vi "Request Message Loop.vi"(8 "error in (no error)":errorcluster, 11 "Message Queues":T1) -> (0 "error out":errorcluster)   [LabVIEW 2023, in "Weather Request Loop.lvlib"]
doc: "A message handler for sending HTTP requests and parsing the response headers. If needed, the handler will prompt the user to log in."
uses:
  Weather Request Loop.lvlib
  support/Message Queue/All Message Queues.ctl
  support/Message Queue/Message Cluster.ctl
  Request Data.ctl
  <vilib>/httpClient/ClientHandle.ctl
  Response Data.ctl
  support/Message Queue/Weather Message Queue.lvlib
  <vilib>/httpClient/LabVIEWHTTPClient.lvlib
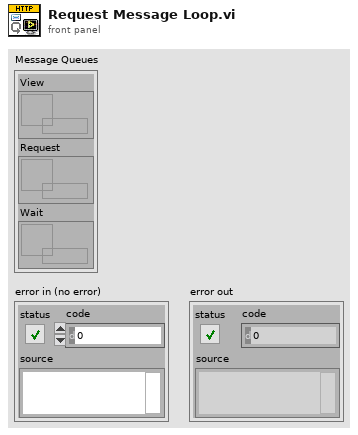
[diagram p1: front panel]
types:
  T1 = typedef "Weather Message Queue.lvlib/All Message Queues.ctl" = cluster{"View":refnum<queue>, "Request":refnum<queue>, "Wait":refnum<queue>}
  T2 = typedef "Weather Request Loop.lvlib/Request Data.ctl" = cluster{"client handle":T3, "URL":string, "Content-Type":string, "Timeout":i32}
  T3 = typedef "LabVIEWHTTPClient.lvlib/ClientHandle.ctl" = refnum<k1>
  T4 = typedef "Weather Request Loop.lvlib/Response Data.ctl" = cluster{"Response Code":u16, "Body":string, "Headers":variant, "error":errorcluster}
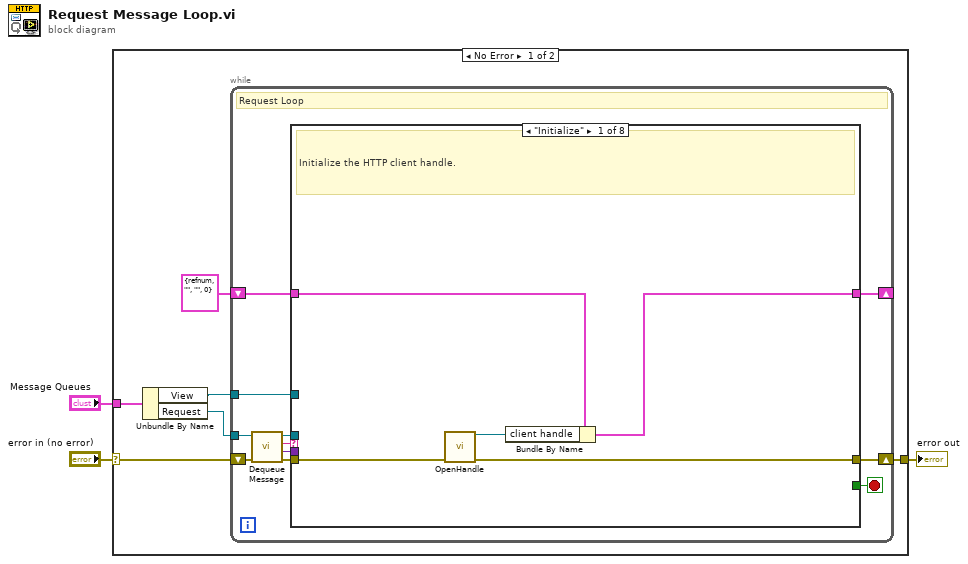
[diagram p0: block diagram]
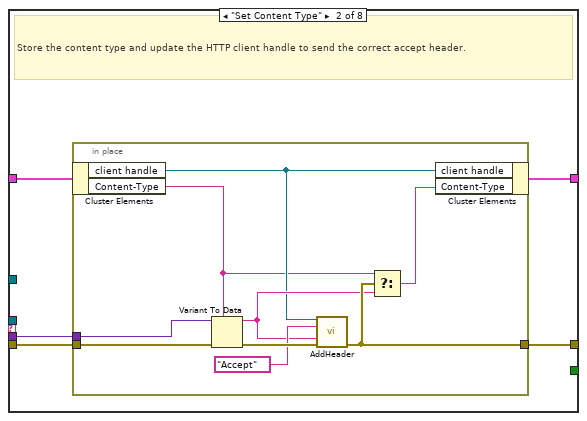
[diagram p2: hidden frame]
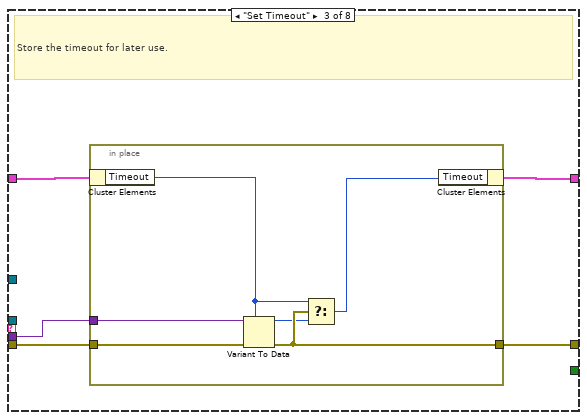
[diagram p3: hidden frame]
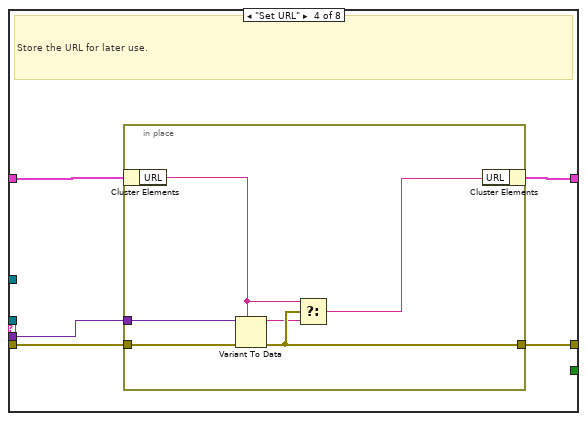
[diagram p4: hidden frame]
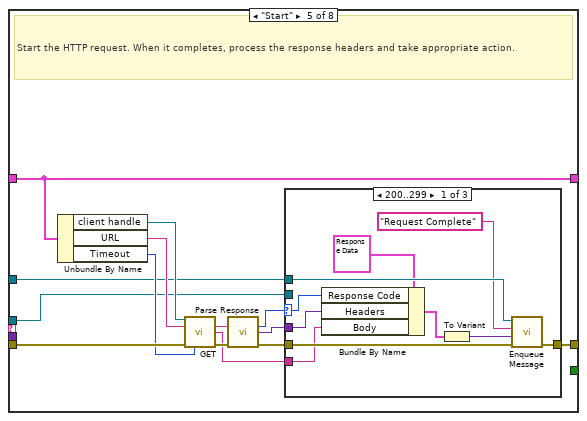
[diagram p5: hidden frame]
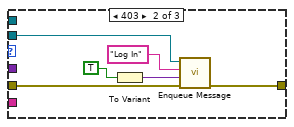
[diagram p6: hidden frame]
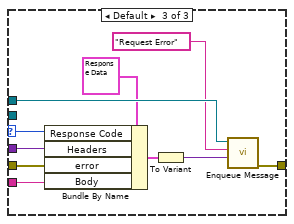
[diagram p7: hidden frame]
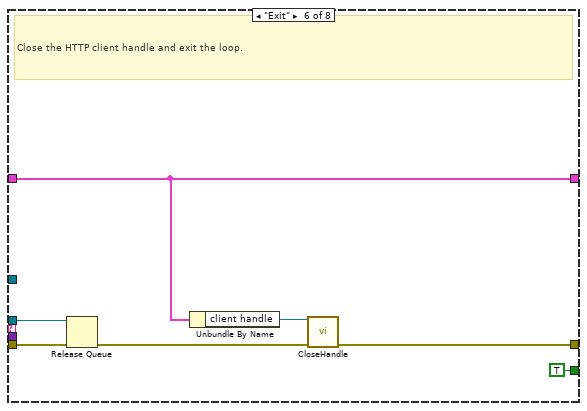
[diagram p8: hidden frame]
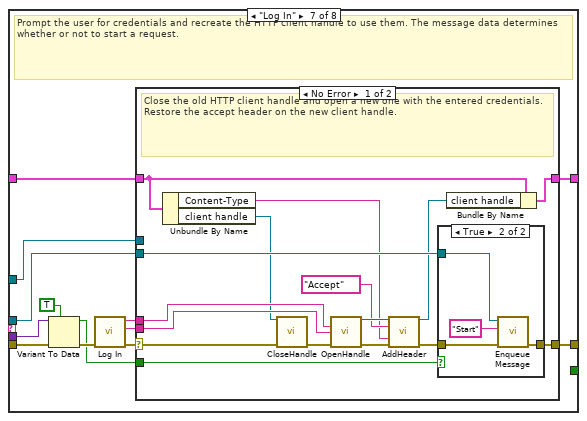
[diagram p9: hidden frame]
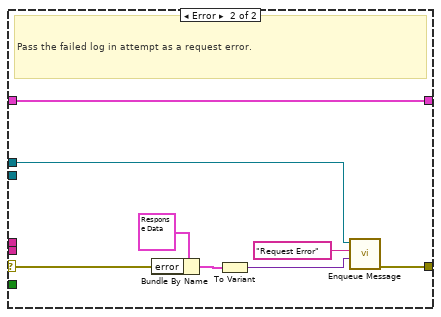
[diagram p11: hidden frame]
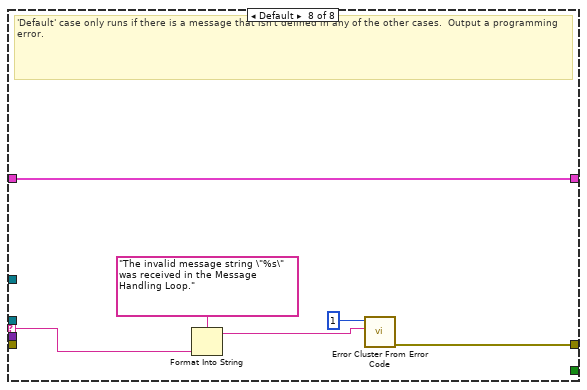
[diagram p12: hidden frame]
diagram:
  n1 = case shown="No Error" "error in (no error)" {
    selector: "error in (no error)" -> [w8 w157]
    tunnel: "Message Queues" -> [w9 _]
    tunnel: [w7 w157] -> w1
    frame No Error {
      n2 = Unbundle By Name(w9) -> ("View"=w6:refnum<queue>, "Request"=w5:refnum<queue>)
      n3 = while {
        shift-right: [w12] -> w7
        shift-left: w8 -> [w19]
        tunnel: w6 -> [w10]
        tunnel: w5 -> [w20]
        shift-right: [w13] -> _
        shift-left: T2 {"client handle"=refnum, "URL"="", "Content-Type"="", "Timeout"=0} ("Request Data") -> [w14]
        stop <- w11 stop-if-true
        # "Request Loop"
        n4 = call "Dequeue Message.vi"("error in (no error)"=w19, "Message Queue"=w20) -> ("error out"=w16:errorcluster, "Message Data"=w15:variant, "Message"=w18:string, "dup Message Queue"=w17:refnum<queue>)  [unwired: 6 in]
        n5 = case shown="\"Initialize\"" w18 {
          selector: w18 -> [_ _ _ _ _ _ _ w151]
          tunnel: w17 -> [_ _ _ _ w63 w102 w113 _]
          tunnel: w16 -> [w25 w30 w44 w55 w75 w108 w121 _]
          tunnel: w15 -> [_ w29 w42 w53 _ _ w111 _]
          tunnel: w14 -> [w24 w27 w41 w52 w74 w105 w117 w156]
          tunnel: [w22 w26 w40 w51 w74 w105 w116 w156] -> w13
          tunnel: [w21 w28 w43 w54 w67 w106 w119 w152] -> w12
          tunnel: [_ _ _ _ _ TRUE _ _] -> w11
          tunnel: w10 -> [_ _ _ _ w65 _ w118 _]
          frame "Initialize" {
            # "Initialize the HTTP client handle."
            n6 = call <vilib>:"OpenHandle.vi"("error in (no error)"=w25) -> ("client handle out"=w23:T3, "error out"=w21:errorcluster)  [unwired: 13 in]
            n7 = Bundle By Name(cluster=w24, "client handle"=w23) -> (w22:T2)
          }
          frame "Set Content Type" {
            # "Store the content type and update the HTTP client handle to send the correct accept header."
            n8 = in-place {
              in-place-border: w30 -> [w39]
              in-place-border: w29 -> [w37]
              in-place-border: [w35] -> w28
              n9 = in-place-cluster #1(w27) -> ("client handle"=w32:T3, "Content-Type"=w31:string)
              n10 = Variant To Data(error in=w39, type=w31, Variant=w37) -> (data=w34:string, error out=w38:errorcluster)
              n11 = call <vilib>:"AddHeader.vi"("client handle"=w32, "header"="Accept", "value"=w34, "error in (no error)"=w38) -> ("error out"=w35:errorcluster)  [unwired: 10 in, 1 out]
              n12 = Select(t=w31, s=w35, f=w34) -> (s? t:f=w33:string)
              n13 = in-place-cluster #1("client handle"=w32, "Content-Type"=w33) -> (w26:T2)
            }
          }
          frame "Set Timeout" {
            # "Store the timeout for later use."
            n14 = in-place {
              in-place-border: w44 -> [w50]
              in-place-border: [w49] -> w43
              in-place-border: w42 -> [w48]
              n15 = in-place-cluster #2(w41) -> ("Timeout"=w46:i32)
              n16 = Variant To Data(error in=w50, type=w46, Variant=w48) -> (data=w47:i32, error out=w49:errorcluster)
              n17 = Select(t=w46, s=w49, f=w47) -> (s? t:f=w45:i32)
              n18 = in-place-cluster #2("Timeout"=w45) -> (w40:T2)
            }
          }
          frame "Set URL" {
            # "Store the URL for later use."
            n19 = in-place {
              in-place-border: w55 -> [w61]
              in-place-border: [w60] -> w54
              in-place-border: w53 -> [w59]
              n20 = in-place-cluster #3(w52) -> ("URL"=w57:string)
              n21 = Variant To Data(error in=w61, type=w57, Variant=w59) -> (data=w58:string, error out=w60:errorcluster)
              n22 = Select(t=w57, s=w60, f=w58) -> (s? t:f=w56:string)
              n23 = in-place-cluster #3("URL"=w56) -> (w51:T2)
            }
          }
          frame "Start" {
            # "Start the HTTP request. When it completes, process the response headers and take appropriate action."
            n24 = Unbundle By Name(w74) -> ("client handle"=w73:T3, "URL"=w72:string, "Timeout"=w71:i32)
            n25 = call <vilib>:"GET.vi"("client handle"=w73, "url"=w72, "error in (no error)"=w75, "timeout (10000)"=w71) -> ("headers"=w70:string, "body"=w62:string, "error out"=w69:errorcluster)  [unwired: 8 in, 1 out]
            n26 = call "Parse Response.vi"("Headers"=w70, "error in (no error)"=w69) -> ("Response code"=w66:u16, "Parsed headers"=w64:variant, "error out"=w68:errorcluster)  [unwired: 11 in]
            n27 = case shown="200..299" w66 {
              selector: w66 -> [w81 _ w95]
              tunnel: w68 -> [w85 w91 w97]
              tunnel: [w84 w90 w101] -> w67
              tunnel: w65 -> [w83 _ w100]
              tunnel: w64 -> [w80 _ w96]
              tunnel: w63 -> [_ w89 _]
              tunnel: w62 -> [w76 _ w92]
              frame 200..299 {
                n28 = Bundle By Name(cluster=T4 {"Response Code"=0, "Body"="", "Headers"=variant, "error"={"status"=FALSE, "code"=0, "source"=""}} ("Response Data"), "Response Code"=w81, "Headers"=w80, "Body"=w76) -> (w79:T4)
                n29 = To Variant(anything=w79) -> (Variant=w78:variant)
                n30 = call "Enqueue Message.vi"("error in (no error)"=w85, "Message Data"=w78, "Message"="Request Complete", "Message Queue"=w83) -> ("error out"=w84:errorcluster)  [unwired: 6 in, 1 out]
              }
              frame 403 {
                n31 = To Variant(anything=TRUE) -> (Variant=w86:variant)
                n32 = call "Enqueue Message.vi"("error in (no error)"=w91, "Message Data"=w86, "Message"="Log In", "Message Queue"=w89) -> ("error out"=w90:errorcluster)  [unwired: 6 in, 1 out]
              }
              frame Default {
                n33 = Bundle By Name(cluster=T4 {"Response Code"=0, "Body"="", "Headers"=variant, "error"={"status"=FALSE, "code"=0, "source"=""}} ("Response Data"), "Response Code"=w95, "Headers"=w96, "error"=w97, "Body"=w92) -> (w94:T4)
                n34 = To Variant(anything=w94) -> (Variant=w93:variant)
                n35 = call "Enqueue Message.vi"("Message Data"=w93, "Message"="Request Error", "Message Queue"=w100) -> ("error out"=w101:errorcluster)  [unwired: 7 in, 1 out]
              }
            }
          }
          frame "Exit" {
            # "Close the HTTP client handle and exit the loop."
            n36 = Release Queue(queue=w102, error in (no error)=w108) -> (error out=w103:errorcluster)  [unwired: 1 in, 2 out]
            n37 = Unbundle By Name(w105) -> ("client handle"=w104:T3)
            n38 = call <vilib>:"CloseHandle.vi"("client handle"=w104, "error in (no error)"=w103) -> ("error out"=w106:errorcluster)  [unwired: 13 in]
          }
          frame "Log In" {
            # "Prompt the user for credentials and recreate the HTTP client handle to use them. The message data determines whether or not to start a request."
            n39 = Variant To Data(error in=w121, type=TRUE, Variant=w111) -> (data=w109:bool, error out=w112:errorcluster)
            n40 = call "Log In.vi"("Error In"=w112) -> ("Error Out"=w120:errorcluster, "Password"=w114:string, "Username"=w115:string)  [unwired: 8 in]
            n41 = case shown="No Error" w120 {
              selector: w120 -> [w136 w148]
              tunnel: [w132 w150] -> w119
              tunnel: w118 -> [_ w146]
              tunnel: w117 -> [w137 w143]
              tunnel: [w131 w143] -> w116
              tunnel: w115 -> [w135 _]
              tunnel: w114 -> [w134 _]
              tunnel: w113 -> [w133 _]
              tunnel: w109 -> [w130 _]
              frame No Error {
                # "Close the old HTTP client handle and open a new one with the entered credentials. Restore the accept header on the new client handle."
                n42 = Unbundle By Name(w137) -> ("Content-Type"=w122:string, "client handle"=w129:T3)
                n43 = call <vilib>:"CloseHandle.vi"("client handle"=w129, "error in (no error)"=w136) -> ("error out"=w128:errorcluster)  [unwired: 13 in]
                n44 = call <vilib>:"OpenHandle.vi"("username"=w135, "password"=w134, "error in (no error)"=w128) -> ("client handle out"=w125:T3, "error out"=w127:errorcluster)  [unwired: 11 in]
                n45 = call <vilib>:"AddHeader.vi"("client handle"=w125, "header"="Accept", "value"=w122, "error in (no error)"=w127) -> ("client handle out"=w124:T3, "error out"=w126:errorcluster)  [unwired: 10 in]
                n46 = case shown="True" w130 {
                  tunnel: w126 -> [w138 w142]
                  tunnel: [w138 w141] -> w132
                  tunnel: w133 -> [_ w140]
                  frame False {
                  }
                  frame True {
                    n47 = call "Enqueue Message.vi"("error in (no error)"=w142, "Message"="Start", "Message Queue"=w140) -> ("error out"=w141:errorcluster)  [unwired: 7 in, 1 out]
                  }
                }
                n48 = Bundle By Name(cluster=w137, "client handle"=w124) -> (w131:T2)
              }
              frame Error {
                # "Pass the failed log in attempt as a request error."
                n49 = Bundle By Name(cluster=T4 {"Response Code"=0, "Body"="", "Headers"=variant, "error"={"status"=FALSE, "code"=0, "source"=""}} ("Response Data"), "error"=w148) -> (w147:T4)
                n50 = To Variant(anything=w147) -> (Variant=w145:variant)
                n51 = call "Enqueue Message.vi"("Message Data"=w145, "Message"="Request Error", "Message Queue"=w146) -> ("error out"=w150:errorcluster)  [unwired: 7 in, 1 out]
              }
            }
          }
          frame Default {
            # "'Default' case only runs if there is a message that isn't defined in any of the other cases.  Output a programming error."
            n52 = Format Into String(format string="The invalid message string \"%s\" was received in the Message Handling Loop." ("Unknown Message Error Text"), w151) -> (resulting string=w153:string)  [unwired: 2 in, 1 out]
            n53 = call <vilib>:"Error Cluster From Error Code.vi"("error message (\"\")"=w153, "error code (0)"=1) -> ("error out"=w152:errorcluster)  [unwired: 7 in]
          }
        }
      }
    }
    frame Error {
    }
  }
  "error out" <- w1
